vi "Get XML Tag Attribute Value.vi"(0 "Element In":refnum<k20>, 5 "Name":string, 11 "error in":errorcluster) -> (4 "Element Out":refnum<k20>, 6 "Value":string, 15 "error out":errorcluster)   [LabVIEW 2016, in "Tree Manager.lvclass"]
uses:
  Tree Manager.lvclass
  <resource>/objmgr/DOMUserDefRef.rc
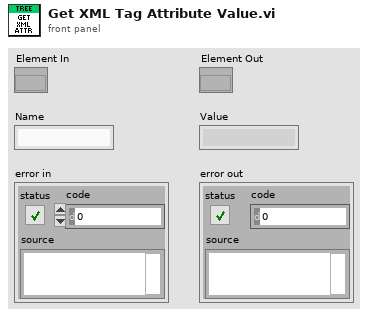
[diagram p1: front panel]
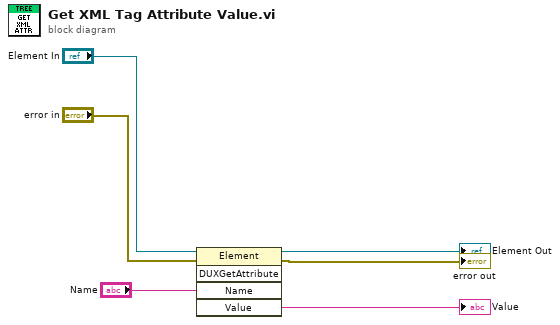
[diagram p0: block diagram]
diagram:
  n1 = invoke class="Element" method="DUXGetAttribute"(reference="Element In", error in="error in", "Name"="Name") -> (reference out=→"Element Out":refnum<k20>, error out=→"error out":errorcluster, "Value"=→"Value":string)  [unwired: 2 in, 2 out]
